vi "SetAalborgServer.vi"(4 "minFlowrate (l/min)":dbl format="%.2f", 5 "Pressure channel":string, 6 "maxFlowrate (l/min)":dbl format="%.2f", 7 "Temperature channel":string, 8 "C:Dem(%)":dbl min=0.0 max=100.0 step=1.0 format="%.2f", 9 "Gas Release System":string, 10 "Q[Total]:Dem(l/min)":dbl format="%.2f", 11 "Mode":T5=enum."Check Flows Are Achievable") -> (1 "WatchChannel":string, 3 "ErrorString":string)   [LabVIEW 2016]
uses:
  Sub VI's/Gas management/CPP/AalborgServerModes.ctl
  Sub VI's/Gas management/CPP/AalborgServerData.ctl
  Sub VI's/Gas management/CPP/MFCdescription.ctl
  Sub VI's/Gas management/CPP/MFCcapability.ctl
  Sub VI's/Gas management/CPP/AalborgServerControlBus.ctl
  Sub VI's/Gas management/CPP/AalborgServerStates.ctl
  ADAM Client/Sub VIs/ADAM Controls/Update_scan_value.ctl
panel:
  out "ControlBus":T1
  out "DataBus":T2
  in  "Tab Control":enum32{"Page 1", "Page 2"}(tab)
  out "Q[Carrier]:Dem(l/min)":dbl
  out "Q[Trace]:Dem(l/min)":dbl
  out "Mdot[Carrier]:Dem(g/min)":dbl
  out "Mdot[Trace]:Dem(g/min)":dbl
  out "Temp:(C)":dbl
  out "Press:(mBar)":dbl
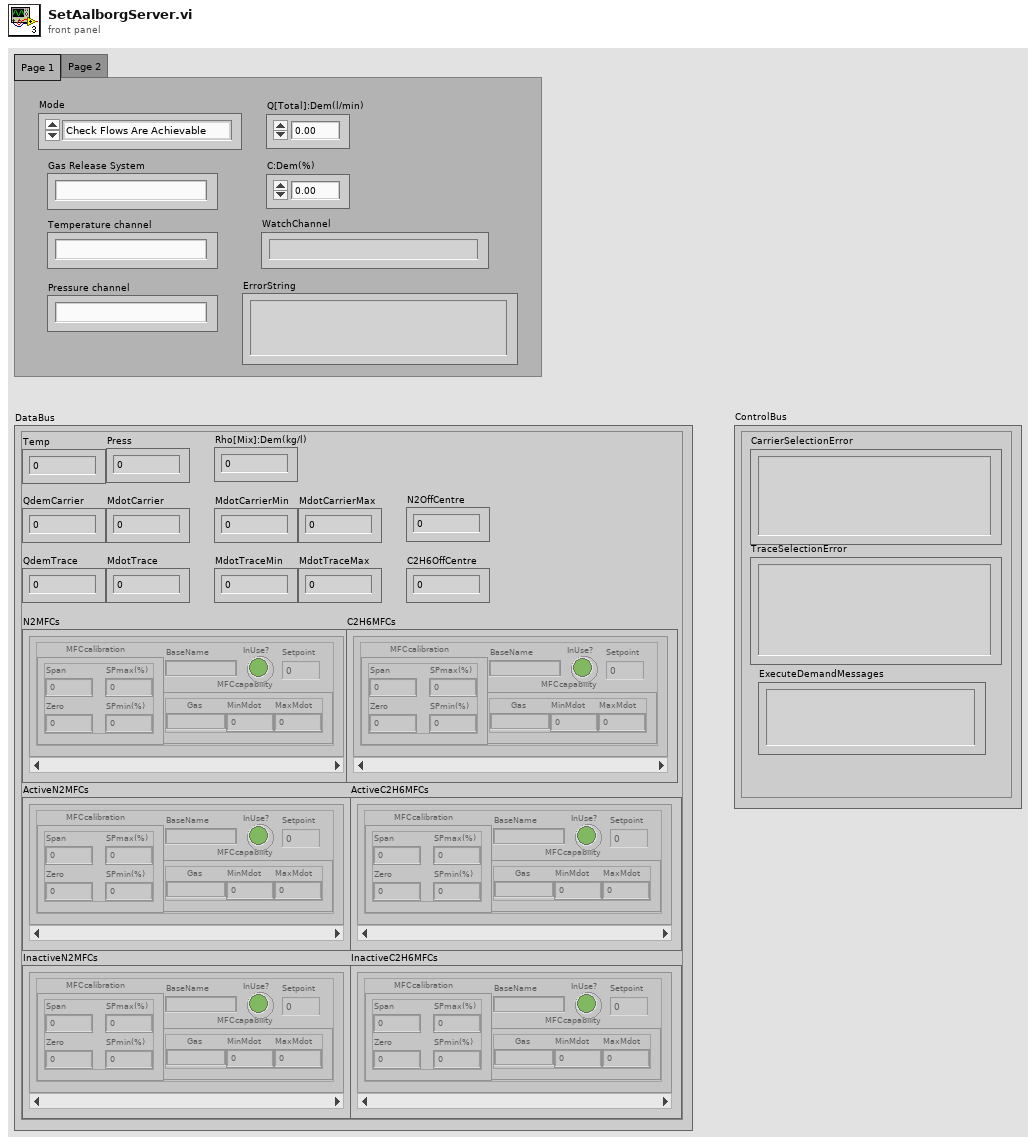
[diagram p1: front panel]
types:
  T1 = typedef "AalborgServerControlBus.ctl" = cluster{"CarrierSelectionError":string, "TraceSelectionError":string, "ExecuteDemandMessages":string}
  T2 = typedef "AalborgServerData.ctl" = cluster{"Temp":dbl, "Press":dbl, "QdemCarrier":dbl, "QdemTrace":dbl, "MdotCarrier":dbl, "MdotCarrierMin":dbl, "MdotCarrierMax":dbl, "MdotTrace":dbl, "MdotTraceMin":dbl, "MdotTraceMax":dbl, "N2MFCs":T3[], "C2H6MFCs":T3[], "N2OffCentre":dbl, "C2H6OffCentre":dbl, "ActiveN2MFCs":T3[], "InactiveN2MFCs":T3[], "ActiveC2H6MFCs":T3[], "InactiveC2H6MFCs":T3[], "Rho[Mix]:Dem(kg/l)":dbl}
  T3 = typedef "MFCdescription.ctl" = cluster{"BaseName":string, "MFCcalibration":cluster{"Span":dbl, "Zero":dbl, "SPmin(%)":dbl, "SPmax(%)":dbl}, "MFCcapability":T4, "InUse?":bool, "Setpoint":dbl}
  T4 = typedef "MFCcapability.ctl" = cluster{"Gas":string, "MinMdot":dbl, "MaxMdot":dbl}
  T5 = typedef "AalborgServerModes.ctl" = enum16{"Set Flows", "Check Flows Are Achievable", "Close All MFCs"}
  T6 = typedef "AalborgServerStates.ctl" = enum16{"Initialise", "Supervise", "ComputeFlowrates", "ADAMiseDemands", "ListMFCchannels", "ChooseMFCs", "CalculateSetpoints", "ExecuteSetpoints", "CloseAll", "Summarise"}
  T7 = enum16{"Append to Global", "Read Global then Clear"}
  T8 = typedef "Update_scan_value.ctl" = cluster{"Channel Name":string, "New Value":dbl}
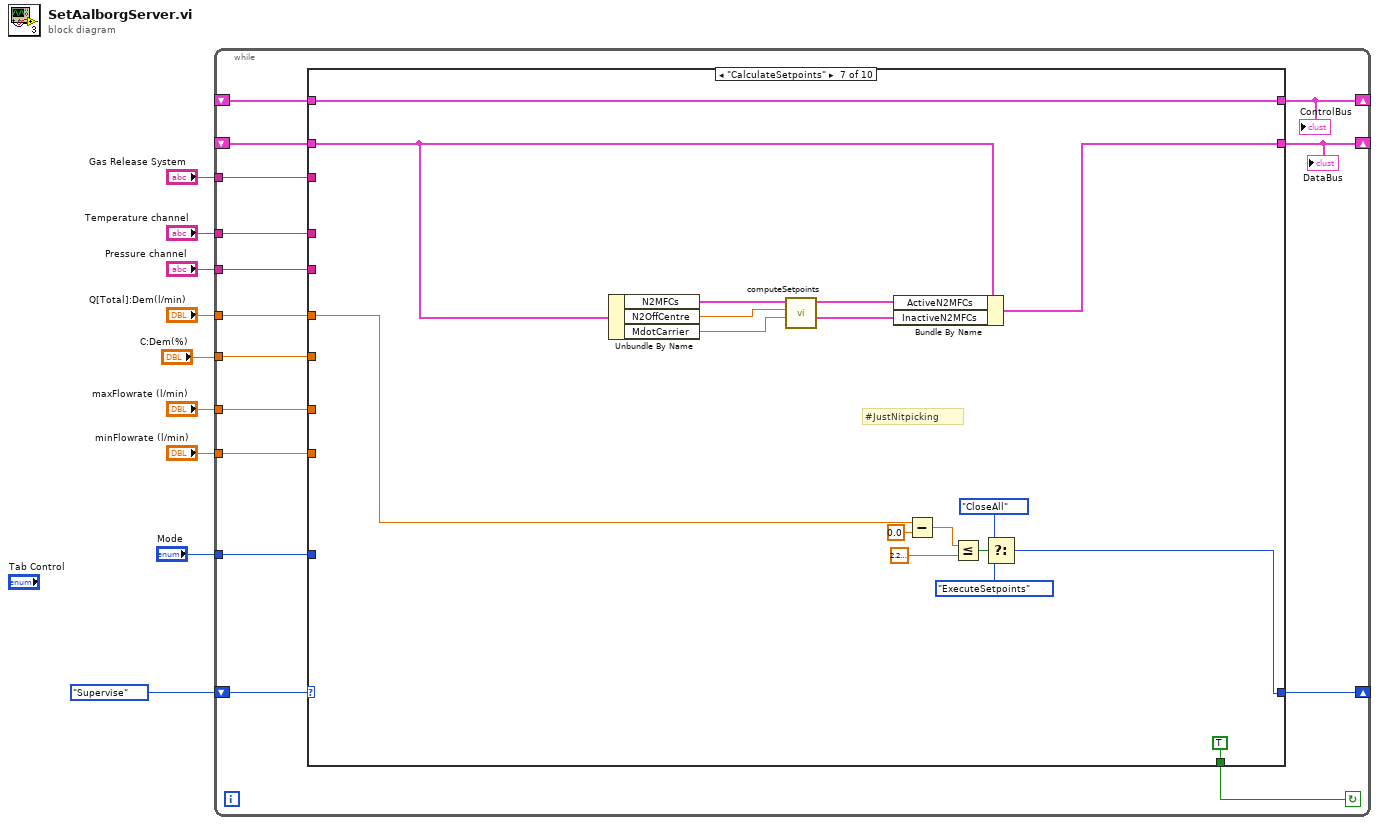
[diagram p0: block diagram]
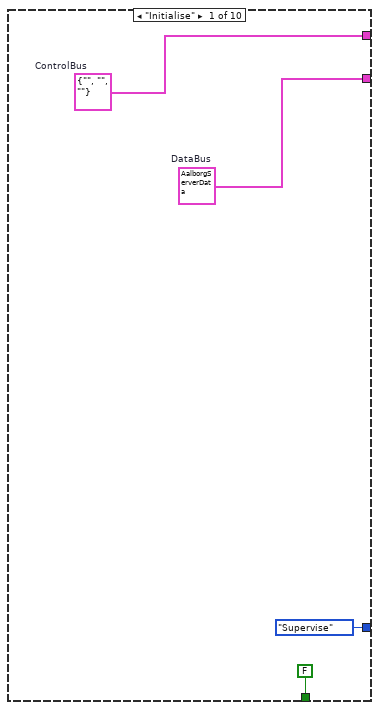
[diagram p2: hidden frame]
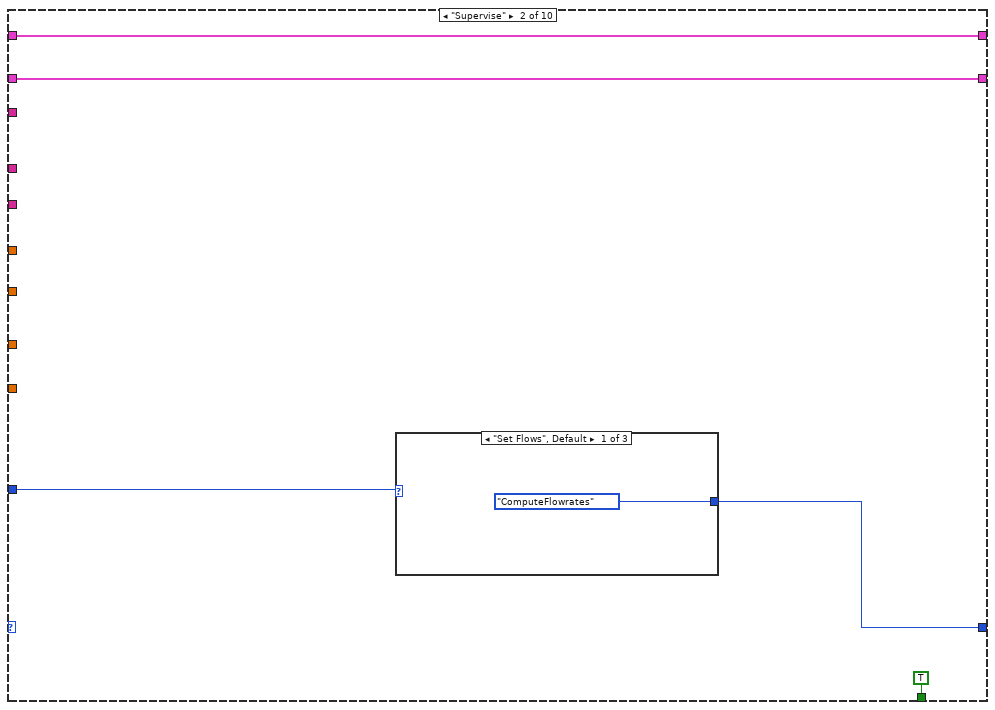
[diagram p3: hidden frame]
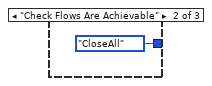
[diagram p4: hidden frame]
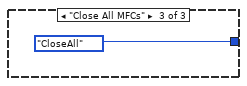
[diagram p5: hidden frame]
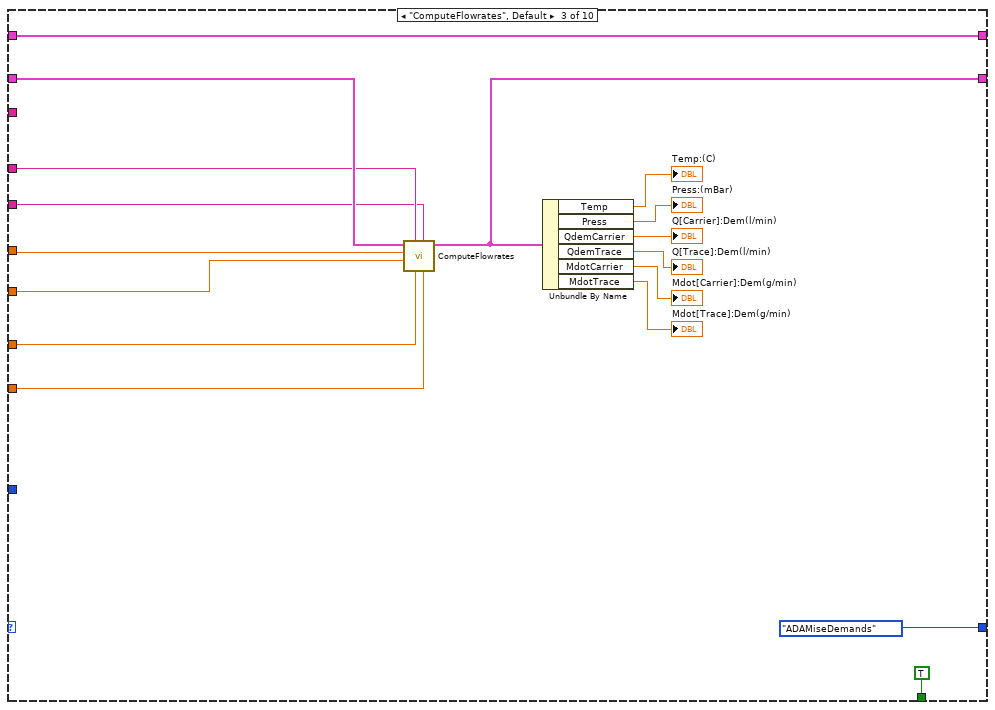
[diagram p6: hidden frame]
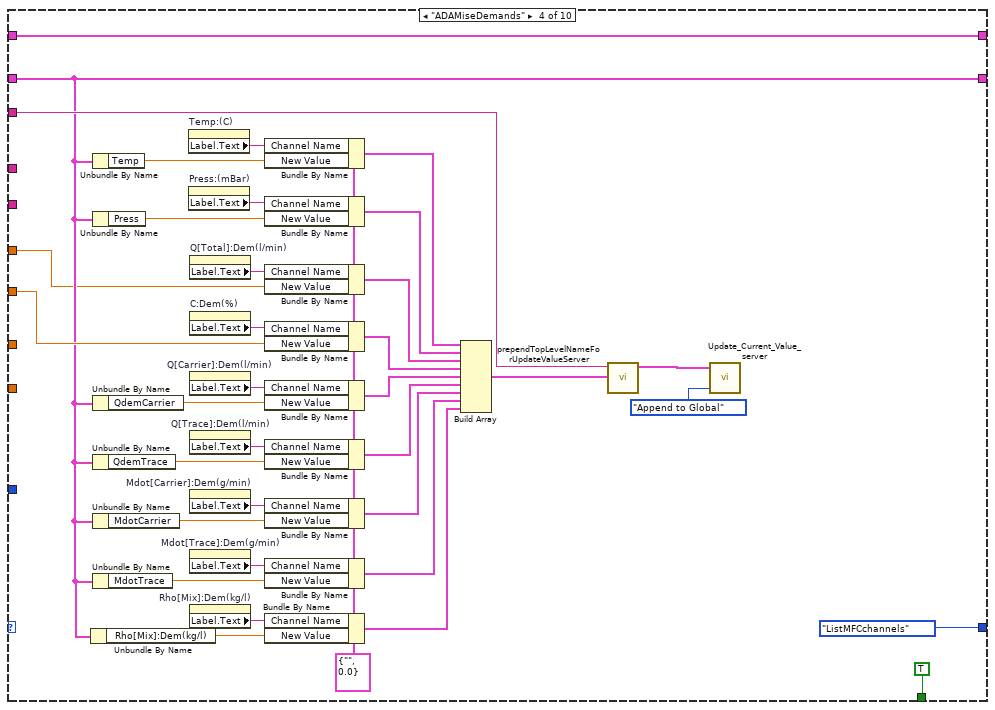
[diagram p7: hidden frame]
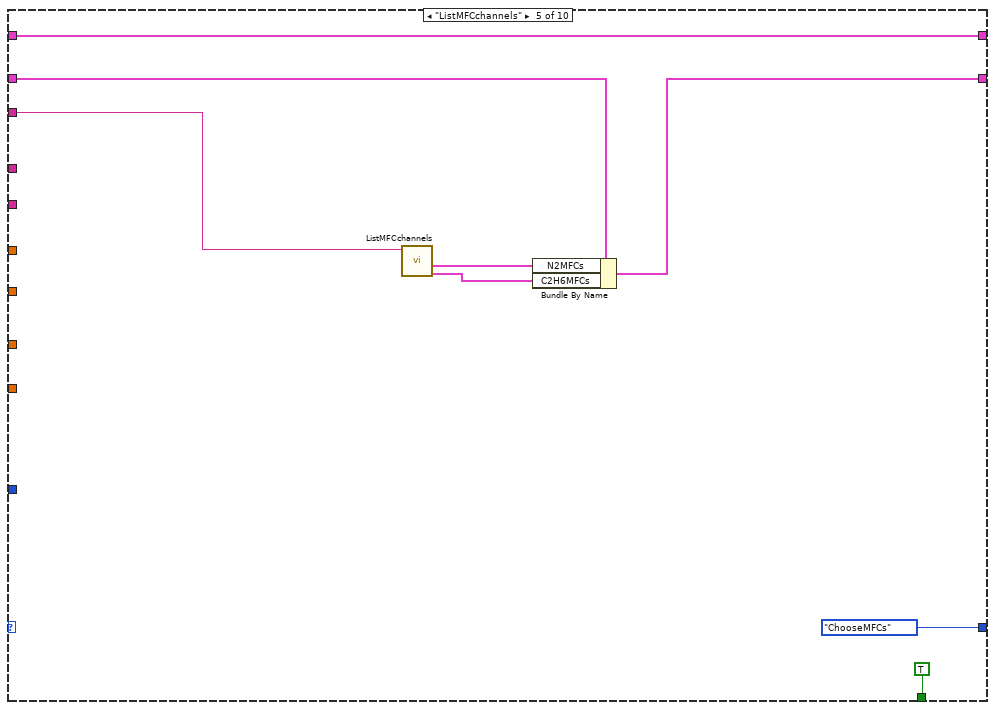
[diagram p8: hidden frame]
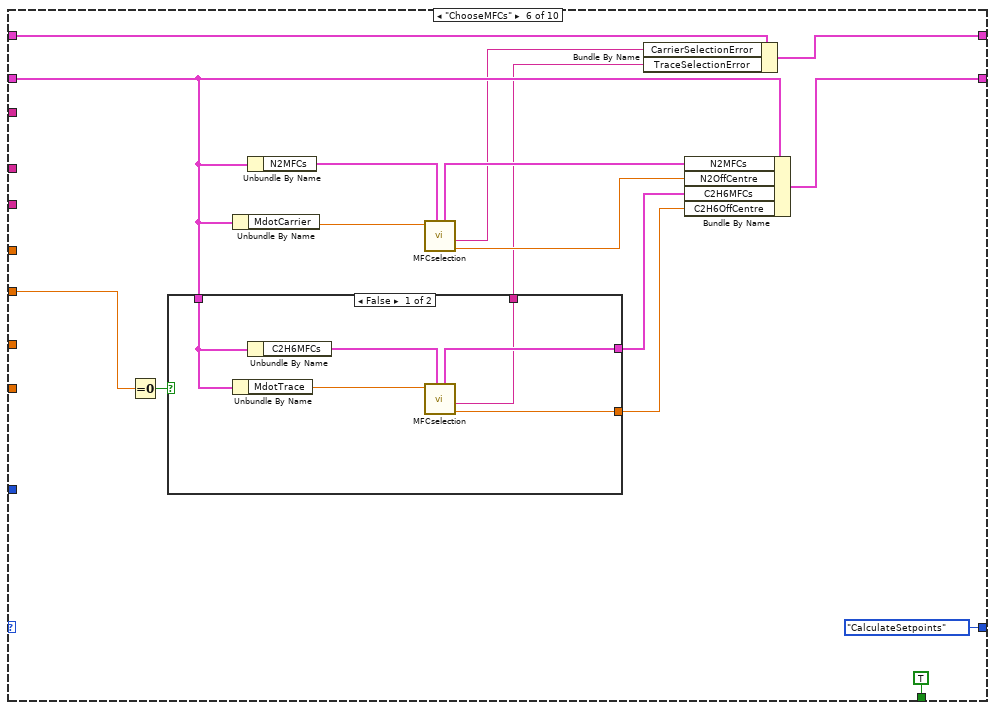
[diagram p9: hidden frame]
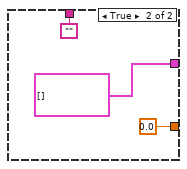
[diagram p10: hidden frame]
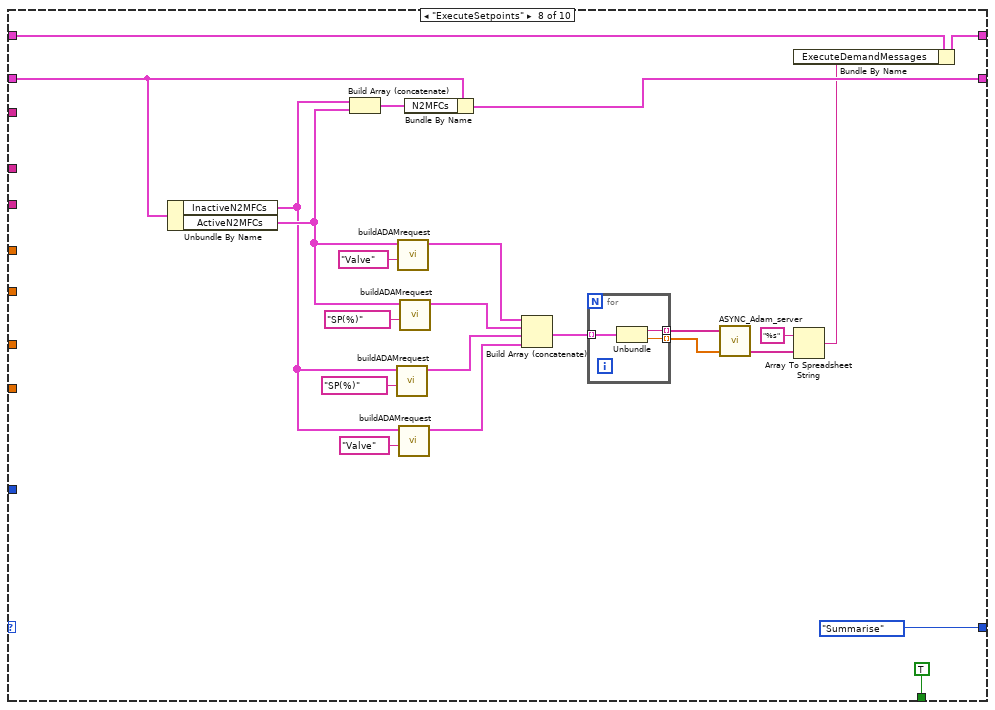
[diagram p11: hidden frame]
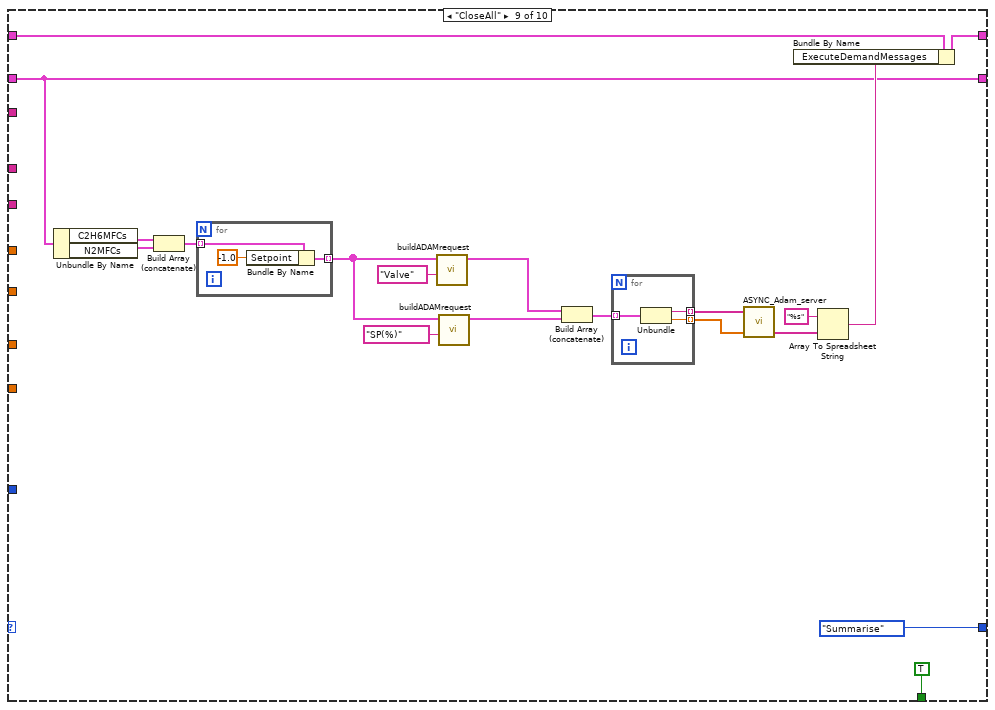
[diagram p12: hidden frame]
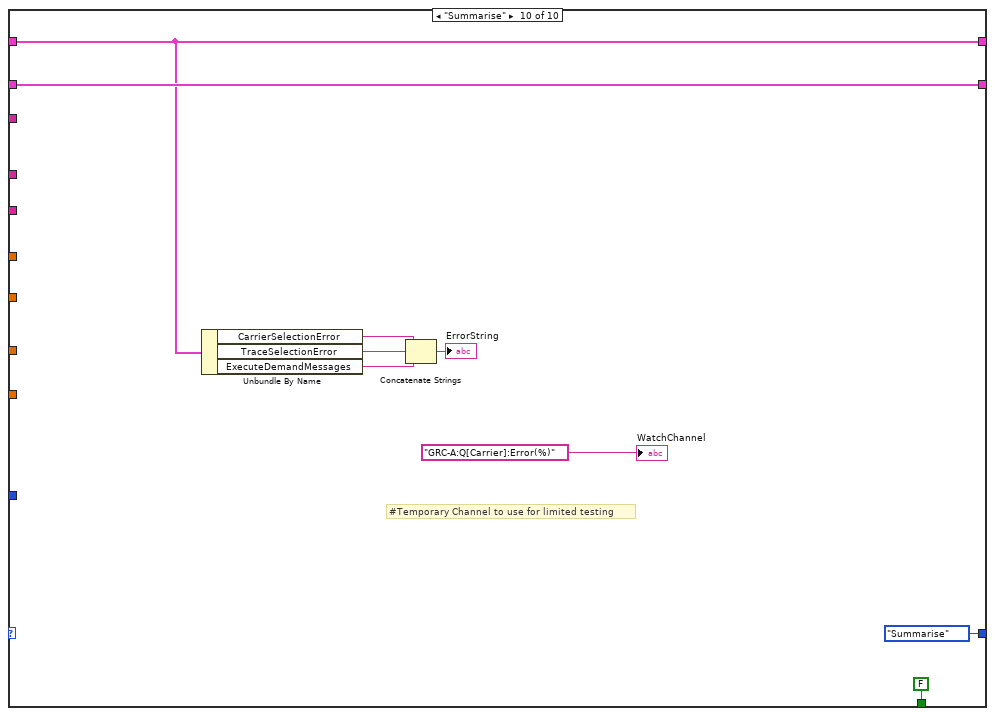
[diagram p13: hidden frame]
diagram:
  n1 = while {
    shift-right: [w23] -> _
    shift-left: _ -> [w22]
    tunnel: "Q[Total]:Dem(l/min)" -> [w24]
    tunnel: "Pressure channel" -> [w20]
    tunnel: "Temperature channel" -> [w19]
    tunnel: "C:Dem(%)" -> [w18]
    shift-right: [w15] -> _
    shift-left: AalborgServerStates."Supervise" -> [w21]
    tunnel: "Gas Release System" -> [w17]
    tunnel: "maxFlowrate (l/min)" -> [w14]
    tunnel: "minFlowrate (l/min)" -> [w13]
    shift-right: [w11] -> _
    shift-left: _ -> [w12]
    tunnel: "Mode" -> [w10]
    stop <- w16 continue-if-true
    n2 = case shown="\"CalculateSetpoints\"" w21 {
      tunnel: w24 -> [_ _ w38 w55 _ _ w126 _ _ _]
      tunnel: [w28 w32 w49 w59 w93 w111 w135 w156 w170 w197] -> w23
      tunnel: w22 -> [_ w32 w53 w59 w94 w110 w136 w157 w170 w197]
      tunnel: w20 -> [_ _ w51 _ _ _ _ _ _ _]
      tunnel: w19 -> [_ _ w52 _ _ _ _ _ _ _]
      tunnel: w18 -> [_ _ w50 w64 _ w107 _ _ _ _]
      tunnel: w17 -> [_ _ _ w63 w97 _ _ _ _ _]
      tunnel: [FALSE TRUE TRUE TRUE TRUE TRUE TRUE TRUE TRUE FALSE] -> w16
      tunnel: [AalborgServerStates."Supervise" w29 AalborgServerStates."ADAMiseDemands" AalborgServerStates."ListMFCchannels" AalborgServerStates."ChooseMFCs" AalborgServerStates."CalculateSetpoints" w129 AalborgServerStates."Summarise" AalborgServerStates."Summarise" AalborgServerStates."Summarise"] -> w15
      tunnel: w14 -> [_ _ w41 _ _ _ _ _ _ _]
      tunnel: w13 -> [_ _ w40 _ _ _ _ _ _ _]
      tunnel: w12 -> [_ w33 w39 w56 w90 w101 w131 w142 w173 w196]
      tunnel: [w25 w33 w39 w56 w90 w100 w131 w141 w172 w196] -> w11
      tunnel: w10 -> [_ w31 _ _ _ _ _ _ _ _]
      frame "Initialise" {
        w25 = T1 {"CarrierSelectionError"="", "TraceSelectionError"="", "ExecuteDemandMessages"=""}  # ControlBus
        w28 = T2 {"Temp"=0.0, "Press"=0.0, "QdemCarrier"=0.0, "QdemTrace"=0.0, "MdotCarrier"=0.0, "MdotCarrierMin"=0.0, "MdotCarrierMax"=0.0, "MdotTrace"=0.0, "MdotTraceMin"=0.0, "MdotTraceMax"=0.0, "N2MFCs"=[], "C2H6MFCs"=[], "N2OffCentre"=0.0, "C2H6OffCentre"=0.0, "ActiveN2MFCs"=[], "InactiveN2MFCs"=[], "ActiveC2H6MFCs"=[], "InactiveC2H6MFCs"=[], "Rho[Mix]:Dem(kg/l)"=0.0}  # DataBus
      }
      frame "Supervise" {
        n3 = case shown="\"Set Flows\", Default" w31 {
          tunnel: [AalborgServerStates."ComputeFlowrates" AalborgServerStates."CloseAll" AalborgServerStates."CloseAll"] -> w29
          frame "Set Flows", Default {
          }
          frame "Check Flows Are Achievable" {
          }
          frame "Close All MFCs" {
          }
        }
      }
      frame "ComputeFlowrates", Default {
        n4 = call "ComputeFlowrates.vi"("minFlowrate (l/min)"=w40, "Pressure channel"=w51, "maxFlowrate (l/min)"=w41, "Temperature channel"=w52, "C_dem:(%)"=w50, "Q_dem[Total]:(l/min)"=w38, "DataBus in"=w53) -> ("DataBus out"=w49:T2)  [unwired: 4 in]
        n5 = Unbundle By Name(w49) -> ("Temp"=→"Temp:(C)":dbl, "Press"=→"Press:(mBar)":dbl, "QdemCarrier"=→"Q[Carrier]:Dem(l/min)":dbl, "QdemTrace"=→"Q[Trace]:Dem(l/min)":dbl, "MdotCarrier"=→"Mdot[Carrier]:Dem(g/min)":dbl, "MdotTrace"=→"Mdot[Trace]:Dem(g/min)":dbl)
      }
      frame "ADAMiseDemands" {
        w58 = T8 {"Channel Name"="", "New Value"=0.0} ("Update Scan Value Cluster")
        n6 = Unbundle By Name(w59) -> ("Rho[Mix]:Dem(kg/l)"=w61:dbl)
        n7 = Unbundle By Name(w59) -> ("Temp"=w70:dbl)
        n8 = Unbundle By Name(w59) -> ("Press"=w69:dbl)
        n9 = Unbundle By Name(w59) -> ("QdemCarrier"=w68:dbl)
        n10 = Unbundle By Name(w59) -> ("QdemTrace"=w67:dbl)
        n11 = Unbundle By Name(w59) -> ("MdotCarrier"=w66:dbl)
        n12 = Unbundle By Name(w59) -> ("MdotTrace"=w65:dbl)
        n13 = property on="Temp:(C)" class="DigNum (strict)"() -> ("Label.Text"=w73:string)  [unwired: 2 in, 2 out]
        n14 = property on="Press:(mBar)" class="DigNum (strict)"() -> ("Label.Text"=w74:string)  [unwired: 2 in, 2 out]
        n15 = property on="Q[Total]:Dem(l/min)" class="DigNum (strict)"() -> ("Label.Text"=w83:string)  [unwired: 2 in, 2 out]
        n16 = property on="C:Dem(%)" class="DigNum (strict)"() -> ("Label.Text"=w82:string)  [unwired: 2 in, 2 out]
        n17 = property on="Q[Carrier]:Dem(l/min)" class="DigNum (strict)"() -> ("Label.Text"=w81:string)  [unwired: 2 in, 2 out]
        n18 = property on="Q[Trace]:Dem(l/min)" class="DigNum (strict)"() -> ("Label.Text"=w80:string)  [unwired: 2 in, 2 out]
        n19 = property on="Mdot[Carrier]:Dem(g/min)" class="DigNum (strict)"() -> ("Label.Text"=w79:string)  [unwired: 2 in, 2 out]
        n20 = property on="Mdot[Trace]:Dem(g/min)" class="DigNum (strict)"() -> ("Label.Text"=w78:string)  [unwired: 2 in, 2 out]
        n21 = property on="Rho[Mix]:Dem(kg/l)" class="DigNum (strict)"() -> ("Label.Text"=w60:string)  [unwired: 2 in, 2 out]
        n22 = Bundle By Name(cluster=w58, "Channel Name"=w73, "New Value"=w70) -> (w71:T8)
        n23 = Bundle By Name(cluster=w58, "Channel Name"=w74, "New Value"=w69) -> (w72:T8)
        n24 = Bundle By Name(cluster=w58, "Channel Name"=w83, "New Value"=w55) -> (w85:T8)
        n25 = Bundle By Name(cluster=w58, "Channel Name"=w82, "New Value"=w64) -> (w86:T8)
        n26 = Bundle By Name(cluster=w58, "Channel Name"=w81, "New Value"=w68) -> (w87:T8)
        n27 = Bundle By Name(cluster=w58, "Channel Name"=w80, "New Value"=w67) -> (w88:T8)
        n28 = Bundle By Name(cluster=w58, "Channel Name"=w79, "New Value"=w66) -> (w89:T8)
        n29 = Bundle By Name(cluster=w58, "Channel Name"=w78, "New Value"=w65) -> (w75:T8)
        n30 = Bundle By Name(cluster=w58, "Channel Name"=w60, "New Value"=w61) -> (w57:T8)
        n31 = Build Array(w71, w72, w85, w86, w87, w88, w89, w75, w57) -> (w77:T8[])
        n32 = call "prependTopLevelNameForUpdateValueServer.vi"("Array in"=w77, "TopLevelADAMname"=w63) -> ("Array out"=w76:T8[])  [unwired: 9 in]
        n33 = call "Update_Current_Value_server.vi"("Mode"=T7."Append to Global", "Update array in"=w76) -> ()  [unwired: 1 in, 1 out]
      }
      frame "ListMFCchannels" {
        n34 = call "ListMFCchannels.vi"("Gas Release System"=w97) -> ("C2H6descriptions"=w91:T3[], "N2descriptions"=w92:T3[])  [unwired: 8 in, 1 out]
        n35 = Bundle By Name(cluster=w94, "N2MFCs"=w92, "C2H6MFCs"=w91) -> (w93:T2)
      }
      frame "ChooseMFCs" {
        n36 = Equal To 0?(x=w107) -> (x = 0?=w108:bool)
        n37 = case shown="False" w108 {
          tunnel: w110 -> [w119 _]
          tunnel: [w116 0.0 ("OffCentre")] -> w103
          tunnel: [w115 T3[] [] ("MFCsOut")] -> w102
          tunnel: [w114 "" ("errorMessage")] -> w98
          frame False {
            n38 = Unbundle By Name(w119) -> ("MdotTrace"=w117:dbl)
            n39 = Unbundle By Name(w119) -> ("C2H6MFCs"=w118:T3[])
            n40 = call "MFCselection.vi"("MFCsIn"=w118, "Mdot"=w117) -> ("OffCentre"=w116:dbl, "errorMessage"=w114:string, "MFCsOut"=w115:T3[])  [unwired: 4 in, 1 out]
          }
          frame True {
          }
        }
        n41 = Unbundle By Name(w110) -> ("MdotCarrier"=w109:dbl)
        n42 = Unbundle By Name(w110) -> ("N2MFCs"=w106:T3[])
        n43 = call "MFCselection.vi"("MFCsIn"=w106, "Mdot"=w109) -> ("OffCentre"=w105:dbl, "errorMessage"=w99:string, "MFCsOut"=w104:T3[])  [unwired: 4 in, 1 out]
        n44 = Bundle By Name(cluster=w101, "CarrierSelectionError"=w99, "TraceSelectionError"=w98) -> (w100:T1)
        n45 = Bundle By Name(cluster=w110, "N2MFCs"=w104, "N2OffCentre"=w105, "C2H6MFCs"=w102, "C2H6OffCentre"=w103) -> (w111:T2)
      }
      frame "CalculateSetpoints" {
        # "#JustNitpicking"
        n46 = Unbundle By Name(w136) -> ("N2MFCs"=w134:T3[], "N2OffCentre"=w138:dbl, "MdotCarrier"=w137:dbl)
        n47 = call "computeSetpoints.vi"("Mdot"=w137, "OffCentre"=w138, "MFCsIn"=w134) -> ("InactiveMFCs 2"=w132:T3[], "ActiveMFCs"=w133:T3[])  [unwired: 7 in]
        n48 = Bundle By Name(cluster=w136, "ActiveN2MFCs"=w133, "InactiveN2MFCs"=w132) -> (w135:T2)
        n49 = Subtract(x=w126, y=0.0) -> (x-y=w124:dbl)
        n50 = Less Or Equal?(x=w124, y=2.220446049250313e-16) -> (x <= y?=w130:bool)
        n51 = Select(t=AalborgServerStates."CloseAll", s=w130, f=AalborgServerStates."ExecuteSetpoints") -> (s? t:f=w129:T6)
      }
      frame "ExecuteSetpoints" {
        n52 = Unbundle By Name(w157) -> ("InactiveN2MFCs"=w150:T3[], "ActiveN2MFCs"=w153:T3[])
        n53 = Build Array (concatenate)(w150, w153) -> (w158:T3[])
        n54 = call "buildADAMrequest.vi"("Aspect"="SP(%)", "MFCs"=w150) -> ("ADAMrequests"=w147:cluster{"String":string, "Setpoint":dbl}[])  [unwired: 9 in]
        n55 = call "buildADAMrequest.vi"("Aspect"="Valve", "MFCs"=w153) -> ("ADAMrequests"=w149:cluster{"String":string, "Setpoint":dbl}[])  [unwired: 9 in]
        n56 = call "buildADAMrequest.vi"("Aspect"="Valve", "MFCs"=w150) -> ("ADAMrequests"=w146:cluster{"String":string, "Setpoint":dbl}[])  [unwired: 9 in]
        n57 = call "buildADAMrequest.vi"("Aspect"="SP(%)", "MFCs"=w153) -> ("ADAMrequests"=w148:cluster{"String":string, "Setpoint":dbl}[])  [unwired: 9 in]
        n58 = Bundle By Name(cluster=w157, "N2MFCs"=w158) -> (w156:T2)
        n59 = Build Array (concatenate)(w149, w148, w147, w146) -> (w145:cluster{"String":string, "Setpoint":dbl}[])
        n60 = for {
          tunnel: w145 -> [w165] mode=indexing
          tunnel: [w164] -> w144 mode=indexing
          tunnel: [w163] -> w143 mode=indexing
          n61 = Unbundle(w165) -> ("String"=w164:string, "Setpoint"=w163:dbl)
        }
        n62 = call "ASYNC_Adam_server.vi"("Values"=w143, "Channel Names"=w144) -> ("Scan Comments"=w159:string[])  [unwired: 2 in, 1 out]
        n63 = Array To Spreadsheet String(array=w159, 3:"%s" ("format string")) -> (spreadsheet string=w140:string)  [unwired: 1 in]
        n64 = Bundle By Name(cluster=w142, "ExecuteDemandMessages"=w140) -> (w141:T1)
      }
      frame "CloseAll" {
        n65 = Unbundle By Name(w170) -> ("C2H6MFCs"=w169:T3[], "N2MFCs"=w166:T3[])
        n66 = Build Array (concatenate)(w169, w166) -> (w167:T3[])
        n67 = for {
          tunnel: w167 -> [w187] mode=indexing
          tunnel: [w185] -> w168 mode=indexing
          n68 = Bundle By Name(cluster=w187, "Setpoint"=-1.0) -> (w185:T3)
        }
        n69 = call "buildADAMrequest.vi"("Aspect"="Valve", "MFCs"=w168) -> ("ADAMrequests"=w178:cluster{"String":string, "Setpoint":dbl}[])  [unwired: 9 in]
        n70 = call "buildADAMrequest.vi"("Aspect"="SP(%)", "MFCs"=w168) -> ("ADAMrequests"=w177:cluster{"String":string, "Setpoint":dbl}[])  [unwired: 9 in]
        n71 = Build Array (concatenate)(w178, w177) -> (w176:cluster{"String":string, "Setpoint":dbl}[])
        n72 = for {
          tunnel: w176 -> [w190] mode=indexing
          tunnel: [w189] -> w175 mode=indexing
          tunnel: [w188] -> w174 mode=indexing
          n73 = Unbundle(w190) -> ("String"=w189:string, "Setpoint"=w188:dbl)
        }
        n74 = call "ASYNC_Adam_server.vi"("Values"=w174, "Channel Names"=w175) -> ("Scan Comments"=w181:string[])  [unwired: 2 in, 1 out]
        n75 = Array To Spreadsheet String(array=w181, 3:"%s" ("format string")) -> (spreadsheet string=w171:string)  [unwired: 1 in]
        n76 = Bundle By Name(cluster=w173, "ExecuteDemandMessages"=w171) -> (w172:T1)
      }
      frame "Summarise" {
        # "#Temporary Channel to use for limited testing"
        n77 = Unbundle By Name(w196) -> ("CarrierSelectionError"=w195:string, "TraceSelectionError"=w194:string, "ExecuteDemandMessages"=w193:string)
        n78 = Concatenate Strings(w195, w194, w193) -> (→"ErrorString":string)
        "WatchChannel" <- "GRC-A:Q[Carrier]:Error(%)"
      }
    }
    "DataBus" <- w23
    "ControlBus" <- w11
  }
